vi "Set message.vi"(10 "WampMessage MsgPack":refnum<class "WampMessage MsgPack.lvclass">, 11 "ErrorHandler MsgPack in":refnum<class "ErrorHandler MsgPack.lvclass">) -> (3 "ErrorHandler MsgPack out":refnum<class "ErrorHandler MsgPack.lvclass">)   [LabVIEW 2020, in "wamplv.lvlib" / "ErrorHandler MsgPack.lvclass"]
uses:
  ErrorHandler MsgPack.lvclass
  ErrorHandler MsgPack.lvclass/ErrorHandler MsgPack.ctl
  SerialisedMessages/MsgPackMessage/WampMessage MsgPack.lvclass
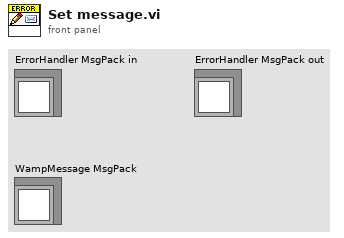
[diagram p1: front panel]
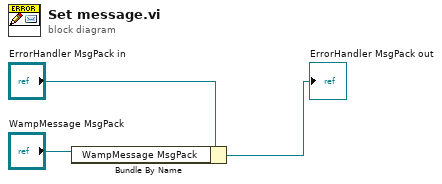
[diagram p0: block diagram]
diagram:
  n1 = Bundle By Name(cluster="ErrorHandler MsgPack in", "WampMessage MsgPack"="WampMessage MsgPack") -> (→"ErrorHandler MsgPack out":refnum<class "ErrorHandler MsgPack.lvclass">)
